vi "串口监视.vi"() -> ()   [LabVIEW 2023]
uses:
  <vilib>/Instr/_visa.llb/VISA Configure Serial Port (Instr).vi
panel:
  out "水泵开关状态":bool
  out "风扇开关状态":bool
  out "光照开关状态":bool
  out "光照":dbl(slide) scale=0.0..100.0
  out "收到的内容":string
  out "土壤湿度":dbl(slide) scale=0.0..100.0
  out "土壤温度":dbl(slide) scale=0.0..100.0
  out "空气湿度":dbl(slide) scale=0.0..100.0
  out "空气温度":dbl(slide) scale=0.0..100.0
  out "错误输出":errorcluster
  in  "开关":bool
  out "状态显示":bool
  in  "VISA resource name":refnum<visa-resource-name> caption="VISA资源名称"
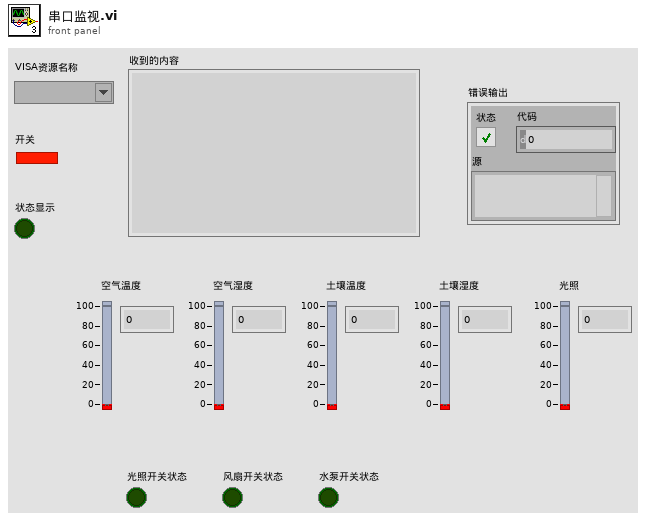
[diagram p1: front panel]
types:
  T1 = enum16{"open", "replace", "create", "open or create", "replace or create", "replace or create with confirmation"}
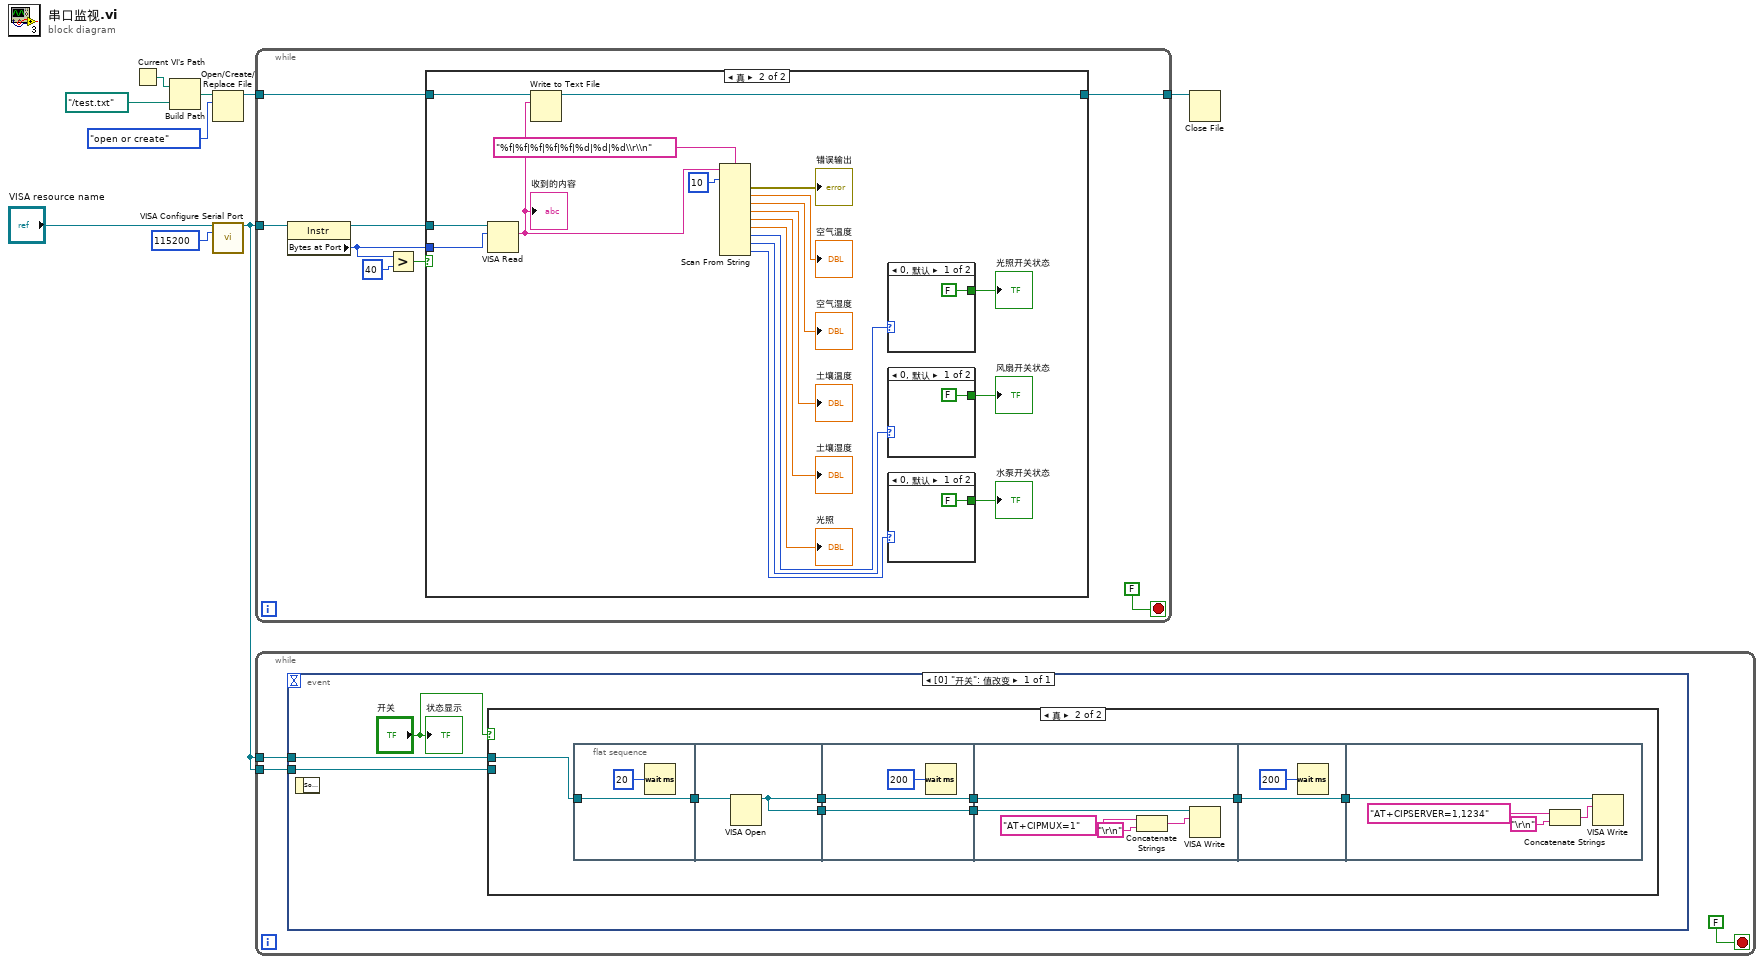
[diagram p0: block diagram]
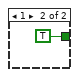
[diagram p3: hidden frame]
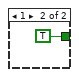
[diagram p4: hidden frame]
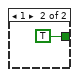
[diagram p5: hidden frame]
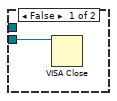
[diagram p6: hidden frame]
diagram:
  n1 = Current VI's Path() -> (path=w4:path)
  n2 = Build Path(base path=w4, name or relative path=path "../test.txt" ("名称或相对路径")) -> (appended path=w5:path)
  n3 = Open/Create/Replace File(file path (use dialog)=w5, operation (0:open)=T1."open or create" ("操作(0:open)")) -> (refnum out=w1:refnum<file>)  [unwired: 4 in, 2 out]
  n4 = call-poly "VISA Configure Serial Port"("VISA resource name"="VISA resource name", "baud rate (9600)"=u32 115200) -> ("VISA resource name out"=w8:refnum<visa-resource-name>)  [unwired: 12 in, 1 out]
  n5 = while {
    tunnel: w8 -> [w12]
    tunnel: [w11] -> w6
    tunnel: w1 -> [w10]
    stop <- FALSE stop-if-true
    n6 = property class="Instr"(reference=w12) -> (reference out=w14:refnum<visa-resource-name>, "Bytes at Port"=w15:u32)  [unwired: 1 in, 1 out]
    n7 = Greater?(x=w15, y=u32 40) -> (0:w16:bool)
    n8 = case shown="真" w16 {
      tunnel: w14 -> [_ w37]
      tunnel: w15 -> [_ w36]
      tunnel: w10 -> [w18 w20]
      tunnel: [w18 w19] -> w11
      frame False {
      }
      frame True {
        n9 = VISA Read(VISA resource name=w37, byte count=w36) -> (read buffer=w21:string)  [unwired: 1 in, 3 out]
        "收到的内容" <- w21
        n10 = Write to Text File(file (use dialog)=w20, text=w21) -> (refnum out=w19:refnum<file>)  [unwired: 2 in, 2 out]
        n11 = Scan From String(format string="%f|%f|%f|%f|%f|%d|%d|%d\\r\\n" ("格式字符串"), input string=w21, initial scan location=u32 10 ("初始扫描位置")) -> (error out=→"错误输出":errorcluster, output 1=→"空气温度":dbl, output 2=→"空气湿度":dbl, output 3=→"土壤温度":dbl, output 4=→"土壤湿度":dbl, output 5=→"光照":dbl, output 6=w27:i32, output 7=w25:i32, output 8=w22:i32)  [unwired: 9 in, 2 out]
        n12 = case shown="0, 默认" w27 {
          tunnel: [FALSE TRUE ("光照开关状态")] -> w26
          frame 0, Default {
          }
          frame 1 {
          }
        }
        "光照开关状态" <- w26
        n13 = case shown="0, 默认" w25 {
          tunnel: [FALSE TRUE ("光照开关状态")] -> w24
          frame 0, Default {
          }
          frame 1 {
          }
        }
        "风扇开关状态" <- w24
        n14 = case shown="0, 默认" w22 {
          tunnel: [FALSE TRUE ("光照开关状态")] -> w23
          frame 0, Default {
          }
          frame 1 {
          }
        }
        "水泵开关状态" <- w23
      }
    }
  }
  n15 = while {
    tunnel: w8 -> [w45]
    tunnel: w8 -> [w44]
    stop <- FALSE stop-if-true
    n16 = event shown="[0] \"开关\": 值改变" {
      selector: _ -> [_]
      dyn-events: _ -> [_]
      timeout: _ -> [_]
      tunnel: w44 -> [w49]
      tunnel: w45 -> [w48]
      event "开关": Value Change {
        n17 = event-data() -> ()  [unwired: 1 in, 1 out]
        n18 = case shown="真" "开关" {
          tunnel: w49 -> [_ w58]
          tunnel: w48 -> [w50 _]
          frame False {
            n19 = VISA Close(VISA resource name=w50) -> ()  [unwired: 1 in, 1 out]
          }
          frame True {
            n20 = flat-sequence {
              tunnel: w58 -> [w60]
              tunnel: [w60] -> w51
              tunnel: [w61] -> w57
              tunnel: [w61] -> w55
              tunnel: w51 -> [w62]
              tunnel: w57 -> [w65]
              tunnel: [w65] -> w56
              tunnel: w55 -> [w63]
              tunnel: [w63] -> w54
              tunnel: w56 -> [w70]
              tunnel: w54 -> [w66]
              tunnel: [w66] -> w53
              tunnel: w53 -> [w71]
              tunnel: [w71] -> w52
              tunnel: w52 -> [w73]
              frame #0 {
                n21 = Wait (ms)(milliseconds to wait=u32 20 ("等待时间（毫秒）")) -> ()  [unwired: 1 out]
              }
              frame #1 {
                n22 = VISA Open(VISA resource name=w62) -> (VISA resource name=w61:refnum<visa-resource-name>)  [unwired: 4 in, 1 out]
              }
              frame #2 {
                n23 = Wait (ms)(milliseconds to wait=u32 200 ("等待时间（毫秒）")) -> ()  [unwired: 1 out]
              }
              frame #3 {
                n24 = Concatenate Strings("AT+CIPMUX=1", "\r\n") -> (w67:string)
                n25 = VISA Write(VISA resource name=w70, write buffer=w67) -> ()  [unwired: 1 in, 3 out]
              }
              frame #4 {
                n26 = Wait (ms)(milliseconds to wait=u32 200 ("等待时间（毫秒）")) -> ()  [unwired: 1 out]
              }
              frame #5 {
                n27 = Concatenate Strings("AT+CIPSERVER=1,1234", "\r\n") -> (w74:string)
                n28 = VISA Write(VISA resource name=w73, write buffer=w74) -> ()  [unwired: 1 in, 3 out]
              }
            }
          }
        }
        "状态显示" <- "开关"
      }
    }
  }
  n29 = Close File(refnum=w6) -> ()  [unwired: 1 in, 2 out]
